vi "ReadJavaFile.vi"(11 "file path (dialog if empty)":path=path "/Users/blagojnikolov/Desktop/@tmp/results.txt") -> (0 "array":dbl[][](array[numeric]) format="%#_2g")   [LabVIEW 2023]
panel:
  out "size(s)":i32[](array[numeric])
  out "substring":string
  out "text":string
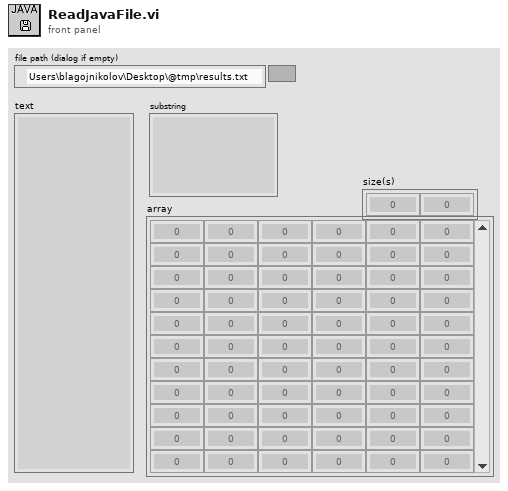
[diagram p1: front panel]
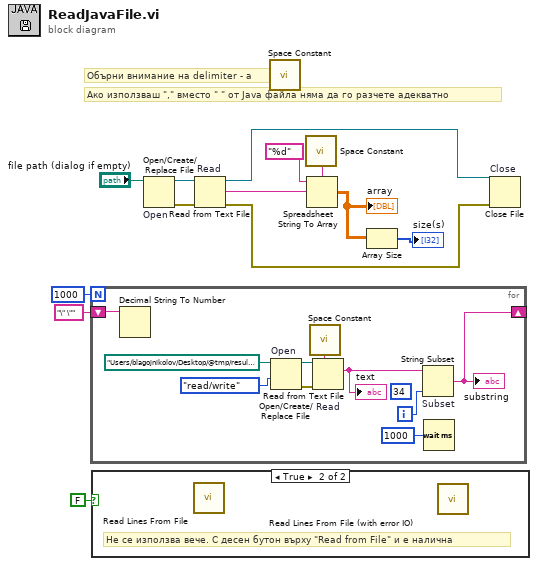
[diagram p0: block diagram]
diagram:
  # "Ако използваш \",\" вместо \" \" от Java файла няма да го разчете адекватно"
  # "Обърни внимание на delimiter - a"
  n1 = for {
    N: 1000 -> [_]
    shift-right: [w14] -> _
    shift-left: "\" \"" -> [w15]
    i -> [w19]
    (unwired) 34 ("length (rest)")
    n2 = Decimal String To Number(string=w15) -> ()  [unwired: 2 in, 2 out]
    n3 = Open/Create/Replace File "Open"(file path (use dialog)=path "/Users/blagojnikolov/Desktop/@tmp/results.txt" ("file path (dialog if empty)"), access (0:read/write)=enum16{"read/write", "read-only", "write-only"}."read/write") -> (refnum out=w21:refnum<file>, error out=w22:errorcluster)  [unwired: 4 in, 1 out]
    n4 = call <vilib>:"Space Constant.vi"() -> ("String"=w17:string)
    n5 = Read from Text File "Read"(prompt (Open existing file)=w17, file (use dialog)=w21, error in=w22) -> (text=w18:string)  [unwired: 1 in, 3 out]
    "text" <- w18
    n6 = String Subset "Subset"(string=w18, length (rest)=w19) -> (substring=w14:string)  [unwired: 1 in]
    "substring" <- w14
    n7 = Wait (ms)(milliseconds to wait=u32 1000) -> ()  [unwired: 1 out]
  }
  n8 = case shown="True" FALSE {
    frame False {
    }
    frame True {
      # "Не се използва вече. С десен бутон върху \"Read from File\" и е налична"
      n9 = call <vilib>:"Read Lines From File.vi"() -> ()  [unwired: 6 in, 4 out]
      n10 = call <vilib>:"Read Lines From File (with error IO).vi"() -> ()  [unwired: 11 in, 5 out]
    }
  }
  n11 = Open/Create/Replace File "Open"(file path (use dialog)="file path (dialog if empty)") -> (refnum out=w11:refnum<file>, error out=w9:errorcluster)  [unwired: 5 in, 1 out]
  n12 = Read from Text File "Read"(file (use dialog)=w11, error in=w9) -> (refnum out=w3:refnum<file>, text=w7:string, error out=w2:errorcluster)  [unwired: 2 in, 1 out]
  n13 = call <vilib>:"Space Constant.vi"() -> ()  [unwired: 1 out]
  n14 = call <vilib>:"Space Constant.vi"() -> ("String"=w8:string)
  n15 = Spreadsheet String To Array(delimiter (Tab)=w8, format string="%d", spreadsheet string=w7) -> (array=w5:dbl[][])  [unwired: 1 in]
  "array" <- w5
  n16 = Array Size(array=w5) -> (size(s)=→"size(s)":i32[])
  n17 = Close File "Close"(refnum=w3, error in=w2) -> ()  [unwired: 2 out]
